vi "set_settings_file.vi"(8 "error in (no error)":errorcluster, 10 "settings cluster in":variant, 11 "StimulatorDL090727DAQmx in":refnum<class "StimulatorDL090727Writer.lvclass">) -> (0 "error out":errorcluster, 3 "StimulatorDL090727DAQmx out":refnum<class "StimulatorDL090727Writer.lvclass">)   [LabVIEW 2010, in "StimulatorDL090727Writer.lvclass"]
uses:
  StimulatorDL090727Writer.lvclass
  StimulatorDL090727Writer.lvclass/StimulatorDL090727Writer.ctl
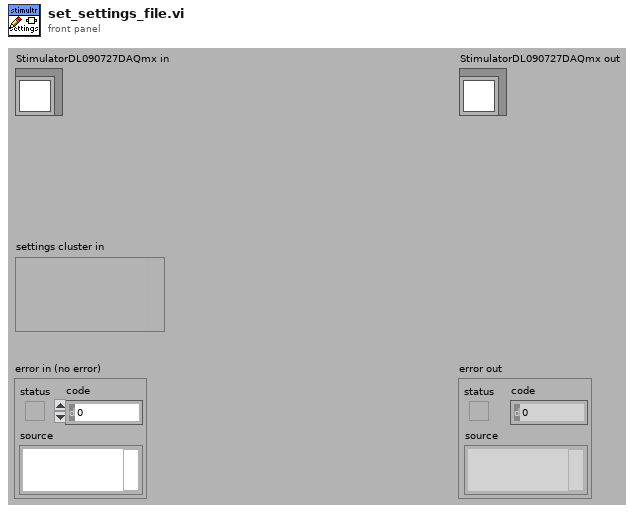
[diagram p1: front panel]
types:
  T1 = typedef "StimulatorDL090727Writer.lvclass/settings_cluster.ctl" = cluster{"Duration":dbl[unit], "Offset":dbl[unit], "DutyCycle":dbl[unit], "Type":T2, "Repetitions":i32, "Frequency":dbl[unit], "Amplitude":dbl}
  T2 = typedef "StimulatorDL090727Writer.lvclass/pattern_enum.ctl" = enum16{"sine wave", "square"}
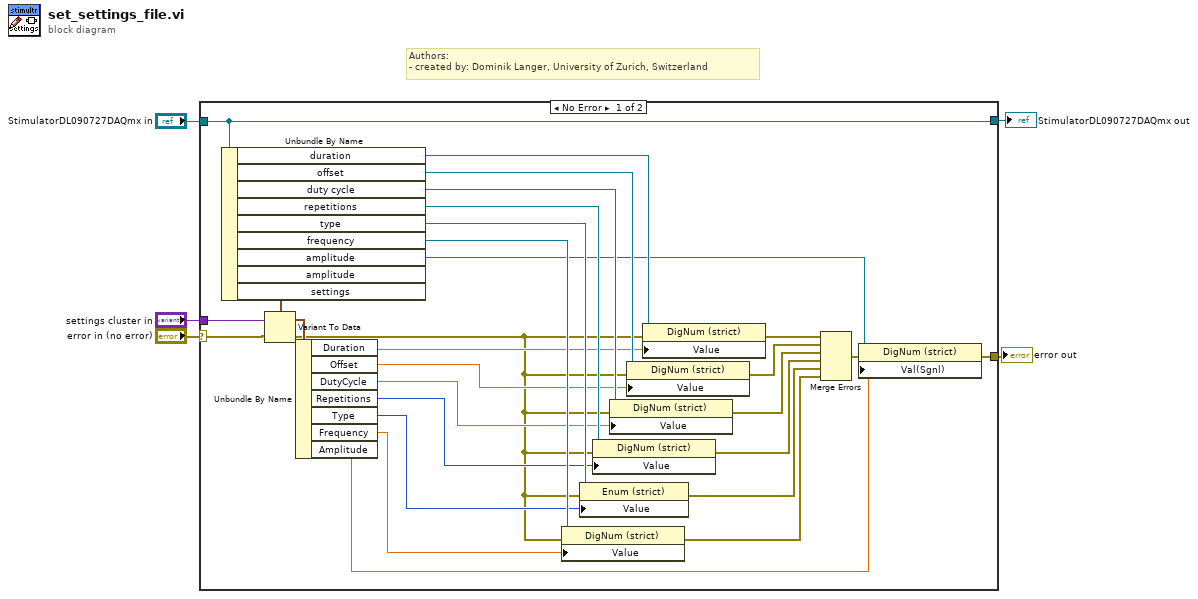
[diagram p0: block diagram]
diagram:
  # "Authors: \n- created by: Dominik Langer, University of Zurich, Switzerland"
  n1 = case shown="No Error" "error in (no error)" {
    selector: "error in (no error)" -> [w14 w34]
    tunnel: "StimulatorDL090727DAQmx in" -> [w11 w35]
    tunnel: [w15 w34] -> w3
    tunnel: [w11 w35] -> w2
    tunnel: "settings cluster in" -> [w13 _]
    frame No Error {
      n2 = Unbundle By Name(w11) -> ("duration"=w32:refnum<vi>, "offset"=w31:refnum<vi>, "duty cycle"=w30:refnum<vi>, "repetitions"=w29:refnum<vi>, "type"=w28:refnum<vi>, "frequency"=w27:refnum<vi>, "amplitude"=w26:refnum<vi>, "settings"=w12:T1)  [unwired: 1 out]
      n3 = Variant To Data(error in=w14, Variant=w13, type=w12) -> (error out=w18:errorcluster, data=w33:T1)
      n4 = Unbundle By Name(w33) -> ("Duration"=w25:dbl[unit], "Offset"=w24:dbl[unit], "DutyCycle"=w23:dbl[unit], "Repetitions"=w22:i32, "Type"=w21:T2, "Frequency"=w20:dbl[unit], "Amplitude"=w19:dbl)
      n5 = property class="DigNum (strict)"(reference=w27, error in=w18, "Value"=w20) -> (error out=w6:errorcluster)  [unwired: 1 out]
      n6 = property class="Enum (strict)"(reference=w28, error in=w18, "Value"=w21) -> (error out=w7:errorcluster)  [unwired: 1 out]
      n7 = property class="DigNum (strict)"(reference=w29, error in=w18, "Value"=w22) -> (error out=w8:errorcluster)  [unwired: 1 out]
      n8 = property class="DigNum (strict)"(reference=w30, error in=w18, "Value"=w23) -> (error out=w9:errorcluster)  [unwired: 1 out]
      n9 = property class="DigNum (strict)"(reference=w31, error in=w18, "Value"=w24) -> (error out=w10:errorcluster)  [unwired: 1 out]
      n10 = property class="DigNum (strict)"(reference=w32, error in=w18, "Value"=w25) -> (error out=w17:errorcluster)  [unwired: 1 out]
      n11 = Merge Errors(w17, w10, w9, w8, w7, w6) -> (w16:errorcluster)
      n12 = property class="DigNum (strict)"(reference=w26, error in=w16, "Val(Sgnl)"=w19) -> (error out=w15:errorcluster)  [unwired: 1 out]
    }
    frame Error {
    }
  }
  "error out" <- w3
  "StimulatorDL090727DAQmx out" <- w2
